vi "AI Reg Set Mapping.vi"(8 "error in (no error)":errorcluster, 10 "Value":u16, 11 "Item Ref in":T1 format="%.0x") -> (0 "error out":errorcluster, 3 "Item Ref out":T1 format="%.0x")   [LabVIEW 2015]
uses:
  <vilib>/NI Veristand/Custom Device API/Custom Device API.lvlib
  Shared/Constants.vi
  Shared/Modbus Master Shared.lvlib
  <vilib>/NI Veristand/Custom Device API/Set Item Property (U16).vi
  <vilib>/NI Veristand/Custom Device API/Custom Device Item Ref.ctl
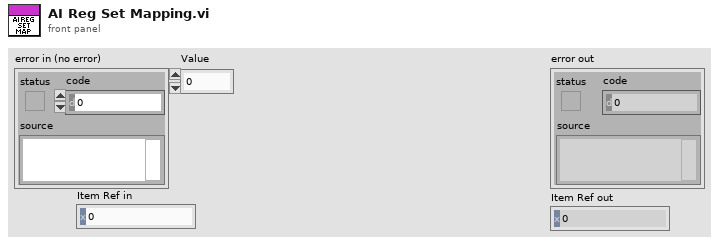
[diagram p1: front panel]
types:
  T1 = typedef "Custom Device API.lvlib/Custom Device Item Ref.ctl" = u64
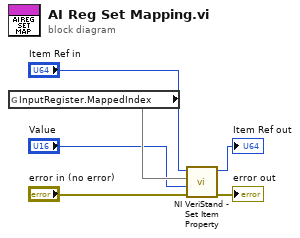
[diagram p0: block diagram]
diagram:
  n1 = global read "Constants.vi" "InputRegister.MappedIndex"() -> (w6)
  n2 = call-poly <vilib>:"NI VeriStand - Set Item Property.vi"("error in (no error)"="error in (no error)", "Value"="Value", "Property Name"=w6, "Item Ref in"="Item Ref in") -> ("error out"=→"error out":errorcluster, "Item Ref out"=→"Item Ref out":T1)  [unwired: 5 in, 1 out]
